vi "Set Step Size Prescale Phase Factor.vi"(8 "error in (no error)":errorcluster, 9 "Step Size Prescale Phase Factor (1)":i32=1, 10 "Prescaler (Output AB)":i32(ring)=1 items=["Output AB"=1, "Output CD"=2, "Output EF"=3, "Output GH"=4], 11 "VISA resource name":refnum<visa-resource-name>) -> (0 "error out":errorcluster, 3 "VISA resource name out":refnum<visa-resource-name>, 4 "Device Errors":cluster{"code":i32, "Text":string}[](array[cluster]))   [LabVIEW 2014, in "Stanford Research DG645 - Driver.lvlib"]
doc: "Trigger Command: SSPH i,j\nInstrument Error Check\n\nSet step size for the prescale phase factor i to j."
uses:
  Stanford Research DG645 - Driver.lvlib
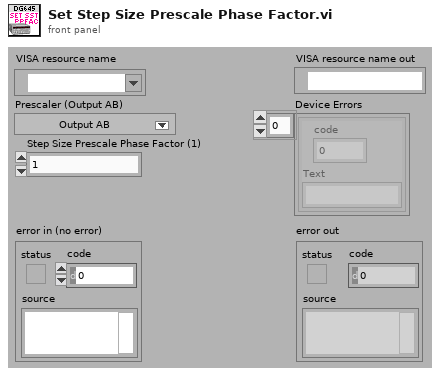
[diagram p1: front panel]
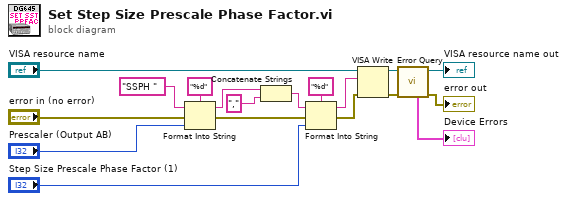
[diagram p0: block diagram]
diagram:
  n1 = Format Into String(format string="%d", initial string="SSPH " ("command"), error in="error in (no error)", "Prescaler (Output AB)") -> (resulting string=w16:string, error out=w17:errorcluster)
  n2 = Concatenate Strings(w16, "," ("command")) -> (w11:string)
  n3 = Format Into String(format string="%d", initial string=w11, error in=w17, "Step Size Prescale Phase Factor (1)") -> (resulting string=w2:string, error out=w1:errorcluster)
  n4 = VISA Write(VISA resource name="VISA resource name", write buffer=w2, error in (no error)=w1) -> (VISA resource name out=w9:refnum<visa-resource-name>, error out=w6:errorcluster)  [unwired: 1 out]
  n5 = call "Error Query.vi"("error in (no error)"=w6, "VISA resource name"=w9) -> ("error out"=→"error out":errorcluster, "VISA resource name out"=→"VISA resource name out":refnum<visa-resource-name>, "Device Errors"=→"Device Errors":cluster{"code":i32, "Text":string}[])  [unwired: 7 in]
